vi "Connect Plugin.vi"(7 "Update Run Pause":bool=TRUE, 8 "error in (no error)":errorcluster, 9 "gRPC ID":T1, 10 "Address":string, 11 "CIF_UI in":refnum<class "CIF_UI.lvclass">) -> (0 "error out":errorcluster, 3 "CIF_UI out":refnum<class "CIF_UI.lvclass">)   [LabVIEW 2021, in "CIF_UI.lvclass"]
uses:
  CIF_UI.lvclass
  <vilib>/gRPC/LabVIEW gRPC Library/Shared/grpcId.ctl
  Typedef/Plugin Connections.ctl
  Typedef/PluginInfo.ctl
  Typedef/Version.ctl
  CIFCore/Common/Typedef/gRPC Reported Plugin Status.ctl
  CIFCore/Common/Typedef/Plugin State.ctl
  CIFCore/Common/Typedef/Timing Statistics.ctl
  CIFCore/Common/Typedef/Timing Stats Base.ctl
  CIFCore/Common/Typedef/FIFO Statistics.ctl
  CIFCore/Common/Typedef/Simple Error.ctl
  CIFCore/Common/Typedef/Monitor Doubles.ctl
  CIFCore/Common/Typedef/Monitor U64.ctl
  CIFCore/Common/Typedef/Monitor I64.ctl
  CIFCore/Common/Typedef/Errors.ctl
  CIF_UI.lvclass/CIF_UI.ctl
  <vilib>/Utility/miscctls.llb/LVMapReplaceAction.ctl
  Accessors/Read Connected.vi
  Accessors/Write IP Address.vi
  Accessors/Write Plugin Connection Map.vi
  Accessors/Read Plugin Connection Map.vi
  Accessors/Write Connected.vi
  <vilib>/CIF Foundation/CIF Utilities/Errors/Append Error Location.vi
  <vilib>/gRPC/LabVIEW gRPC Library/grpc-lvsupport-release.lvlib
  CIFCore/Common/CIFCoreCommon.lvlib
  CIFCore/Grpc/CIFCoreWrapper/CIFCoreWrapper.lvlib
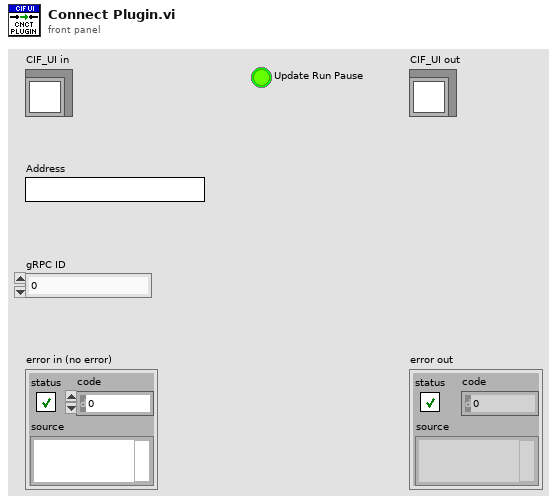
[diagram p1: front panel]
types:
  T1 = typedef "grpc-lvsupport-release.lvlib/grpcId.ctl" = u64
  T2 = typedef "CIF_UI.lvclass/Plugin Connections.ctl" = cluster{"gRPC ID":T1, "Plugin Info":T3}
  T3 = typedef "CIF_UI.lvclass/PluginInfo.ctl" = cluster{"Name":string, "Type":string, "grpc_port":i32, "Version":T4, "Node Status":T5}
  T4 = typedef "CIF_UI.lvclass/Version.ctl" = cluster{"Major":i32, "Minor":i32, "Fix":i32}
  T5 = typedef "CIFCoreCommon.lvlib/gRPC Reported Plugin Status.ctl" = cluster{"State":T6, "Timing Statistics (us)":T7, "FIFO Statistics (us)":T9, "error":T10, "Monitor Doubles":T11, "Monitor U64":T12, "Monitor I64":T13}
  T6 = typedef "CIFCoreCommon.lvlib/Plugin State.ctl" = enum32{"Null", "Creating", "Listening", "Running", "CleaningUp", "Destroying"}
  T7 = typedef "CIFCoreCommon.lvlib/Timing Statistics.ctl" = cluster{"Period":T8, "Wake Error":T8, "Execute":T8, "Housekeep":T8, "Idle":T8, "Cleanup":T8, "Custom 1 (custom units)":T8, "Custom 2 (custom units)":T8}
  T8 = typedef "CIFCoreCommon.lvlib/Timing Stats Base.ctl" = cluster{"Max":i64, "Avg":dbl, "Min":i64}
  T9 = typedef "CIFCoreCommon.lvlib/FIFO Statistics.ctl" = cluster{"From T0":T8, "From Previous Plugin":T8, "Output Error":T8}
  T10 = typedef "CIFCoreCommon.lvlib/Simple Error.ctl" = cluster{"status":bool, "code":i32}
  T11 = typedef "CIFCoreCommon.lvlib/Monitor Doubles.ctl" = cluster{"1":dbl, "2":dbl, "3":dbl, "4":dbl}
  T12 = typedef "CIFCoreCommon.lvlib/Monitor U64.ctl" = cluster{"1":u64, "2":u64, "3":u64, "4":u64}
  T13 = typedef "CIFCoreCommon.lvlib/Monitor I64.ctl" = cluster{"1":i64, "2":i64, "3":i64, "4":i64}
  T14 = typedef "CIFCoreCommon.lvlib/Errors.ctl" = enum16{"Invalid Clock ID", "Long Sleep", "gRPC Server Not Found", "Config Parse", "Timestamp Wrap", "Delayed Execution", "Duplicate Channel", "Missing Channel", "Incorrect Type", "Flatten Error", "Unflatten Data", "Unique Name", "Plugin Not Found", "Plugin Type Not Found", "Plugin Version Not Found", "Manager Not Found", "Numerical Issue", "Time Jump", "Clock ID Match", "Channel Length", "Plugin Connection", "gRPC Server Connection", "PPL Name Match", "Build", "Config Log Parse", "Plugin Load", "UI Subpanel Load", "Python Name", "Invalid Name", "Unable to Change Ch Buffer"}
  T15 = typedef "LVMapReplaceAction.ctl" = enum32{"Modify Entry only if found", "Add or Modify Entry", "Delete Entry"}
  T16 = cluster{"Plugin Name":string, "Plugin Type":string}
  T17 = typedef "CIFCoreCommon.lvlib/Version.ctl" = cluster{"Major":i32, "Minor":i32, "Fix":i32, "Build":i32}
  T18 = typedef "CIF_UI.lvclass/Plugin Connection Map.ctl" = map{string, T2}
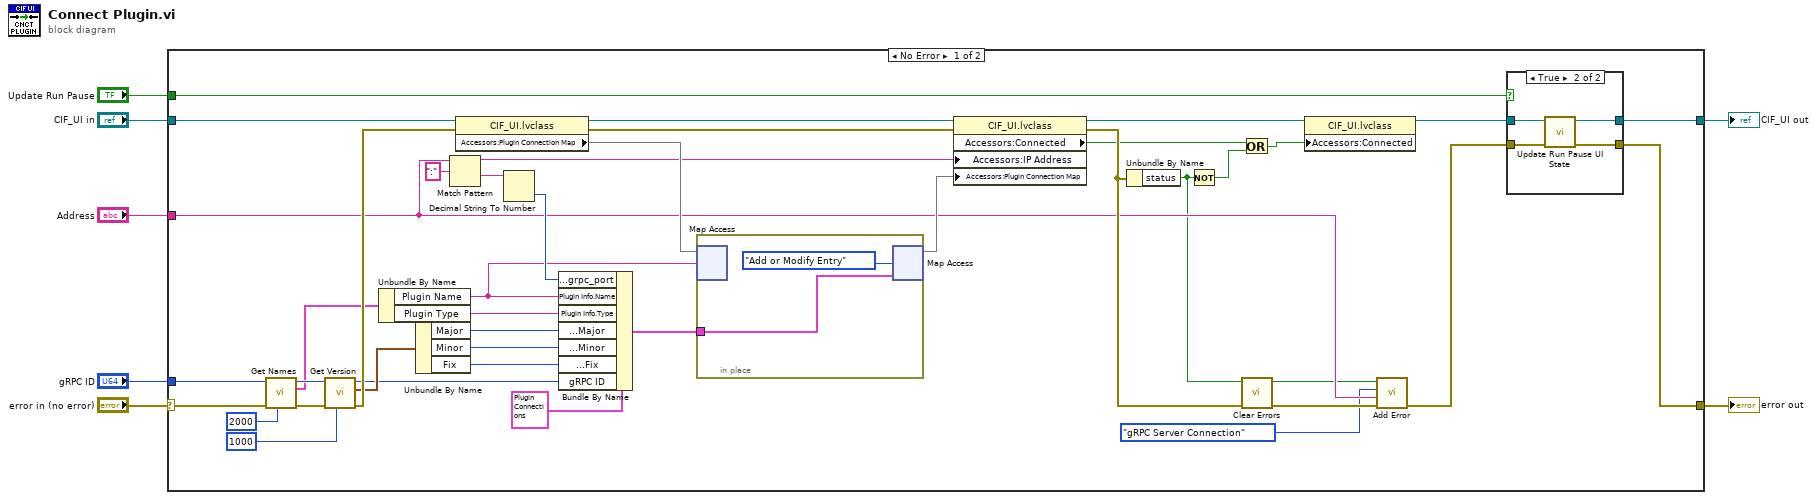
[diagram p0: block diagram]
diagram:
  n1 = case shown="No Error" "error in (no error)" {
    selector: "error in (no error)" -> [w17 w57]
    tunnel: [w21 w57] -> w6
    tunnel: [w22 w56] -> w4
    tunnel: "CIF_UI in" -> [w45 w56]
    tunnel: "Address" -> [w10 _]
    tunnel: "Update Run Pause" -> [w23 _]
    tunnel: "gRPC ID" -> [w16 _]
    frame No Error {
      n2 = call "Get Names.vi"("timeout (ms)"=2000, "error in"=w17, "gRPC ID"=w16) -> ("error out"=w36:errorcluster, "Plugin Names"=w33:T16, "gRPC ID out"=w37:T1)  [unwired: 6 in]
      n3 = call "Get Version.vi"("timeout (ms)"=1000, "error in"=w36, "gRPC ID"=w37) -> ("error out"=w41:errorcluster, "Version"=w20:T17, "gRPC ID out"=w13:T1)  [unwired: 6 in]
      n4 = Unbundle By Name(w33) -> ("Plugin Name"=w28:string, "Plugin Type"=w27:string)
      n5 = Unbundle By Name(w20) -> ("Major"=w19:i32, "Minor"=w18:i32, "Fix"=w15:i32)
      n6 = Match Pattern(string=w10, regular expression=":") -> (before substring=w31:string, after substring=w30:string)  [unwired: 1 in, 2 out]
      n7 = property class="CIF_UI.lvclass"(reference=w45, error in=w41) -> (reference out=w44:refnum<class "CIF_UI.lvclass">, error out=w40:errorcluster, "Accessors:Plugin Connection Map"=w43:T18)
      n8 = Decimal String To Number(string=w30) -> (number=w29:i32)  [unwired: 2 in, 1 out]
      n9 = Bundle By Name(cluster=T2 {"gRPC ID"=0, "Plugin Info"={"Name"="", "Type"="", "grpc_port"=0, "Version"={"Major"=0, "Minor"=0, "Fix"=0}, "Node Status"={"State"=enum."Null", "Timing Statistics (us)"={"Period"={"Max"=0, "Avg"=0.0, "Min"=0}, "Wake Error"={"Max"=0, "Avg"=0.0, "Min"=0}, "Execute"={"Max"=0, "Avg"=0.0, "Min"=0}, "Housekeep"={"Max"=0, "Avg"=0.0, "Min"=0}, "Idle"={"Max"=0, "Avg"=0.0, "Min"=0}, "Cleanup"={"Max"=0, "Avg"=0.0, "Min"=0}, "Custom 1 (custom units)"={"Max"=0, "Avg"=0.0, "Min"=0}, "Custom 2 (custom units)"={"Max"=0, "Avg"=0.0, "Min"=0}}, "FIFO Statistics (us)"={"From T0"={"Max"=0, "Avg"=0.0, "Min"=0}, "From Previous Plugin"={"Max"=0, "Avg"=0.0, "Min"=0}, "Output Error"={"Max"=0, "Avg"=0.0, "Min"=0}}, "error"={"status"=FALSE, "code"=0}, "Monitor Doubles"={"1"=0.0, "2"=0.0, "3"=0.0, "4"=0.0}, "Monitor U64"={"1"=0, "2"=0, "3"=0, "4"=0}, "Monitor I64"={"1"=0, "2"=0, "3"=0, "4"=0}}}} ("value"), "Plugin Info.grpc_port"=w29, "Plugin Info.Name"=w28, "Plugin Info.Type"=w27, "Plugin Info.Version.Major"=w19, "Plugin Info.Version.Minor"=w18, "Plugin Info.Version.Fix"=w15, "gRPC ID"=w13) -> (w42:T2)
      n10 = in-place {
        in-place-border: w42 -> [w55]
        n11 = in-place-map #1(w43, w28) -> ()  [unwired: 1 in, 2 out]
        n12 = in-place-map #1(w55, LVMapReplaceAction."Add or Modify Entry" ("action")) -> (w32:T18)  [unwired: 2 out]
      }
      n13 = property class="CIF_UI.lvclass"(reference=w44, error in=w40, "Accessors:IP Address"=w31, "Accessors:Plugin Connection Map"=w32) -> (reference out=w39:refnum<class "CIF_UI.lvclass">, error out=w38:errorcluster, "Accessors:Connected"=w26:bool)
      n14 = Unbundle By Name(w38) -> ("status"=w8:bool)
      n15 = Not(x=w8) -> (.not. x?=w25:bool)
      n16 = Or(x=w26, y=w25) -> (x .or. y?=w24:bool)
      n17 = call <vilib>:"Clear Errors.vi"("error in (no error)"=w38) -> ("error out"=w12:errorcluster)  [unwired: 5 in, 1 out]
      n18 = property class="CIF_UI.lvclass"(reference=w39, "Accessors:Connected"=w24) -> (reference out=w14:refnum<class "CIF_UI.lvclass">)  [unwired: 1 in, 1 out]
      n19 = call "Add Error.vi"("error in (no error)"=w12, "String to Append"=w10, "Error"=Errors."gRPC Server Connection", "Insert Error"=w8) -> ("error out"=w11:errorcluster)  [unwired: 7 in]
      n20 = case shown="True" w23 {
        tunnel: w11 -> [w48 w52]
        tunnel: w14 -> [w49 w53]
        tunnel: [w49 w50] -> w22
        tunnel: [w48 w51] -> w21
        frame False {
        }
        frame True {
          n21 = call "Update Run Pause UI State.vi"("error in (no error)"=w52, "CIF_UI in"=w53) -> ("error out"=w51:errorcluster, "CIF_UI out"=w50:refnum<class "CIF_UI.lvclass">)  [unwired: 8 in]
        }
      }
    }
    frame Error {
    }
  }
  "error out" <- w6
  "CIF_UI out" <- w4
